vi "Save.vi"(0 "User Configuration Manager in":refnum<class "User Configuration Manager.lvclass">, 5 "Path":path, 11 "error in (no error)":errorcluster, 12 "Persistence":refnum<class "IPersist.lvclass">) -> (4 "User Configuration Manager out":refnum<class "User Configuration Manager.lvclass">, 15 "error out":errorcluster)   [LabVIEW 2017, in "User Configuration Manager.lvlib" / "User Configuration Manager.lvclass"]
doc: "Saves the manager."
uses:
  User Configuration Manager.lvclass
  <vilib>/gpm_packages/@cs/persistence/source/IPersist/IPersist.lvclass
  User Configuration Manager.lvclass/User Configuration Manager.ctl
  Accessors/Read Linked List Ref .vi
  <vilib>/gpm_packages/@cs/linked-list/Source/Linked List/ILinkedList/ILinked List.lvclass
  <vilib>/gpm_packages/@cs/linked-list/Source/Linked List/Linked List Ref/Linked List Ref.lvclass
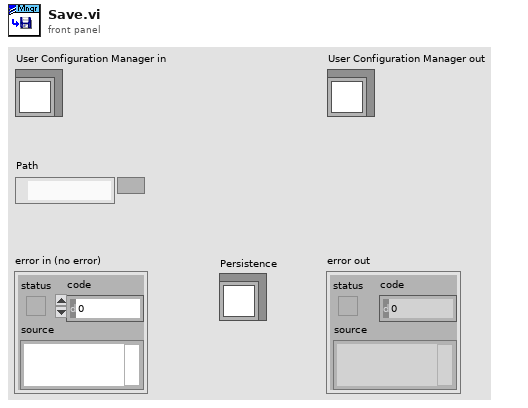
[diagram p1: front panel]
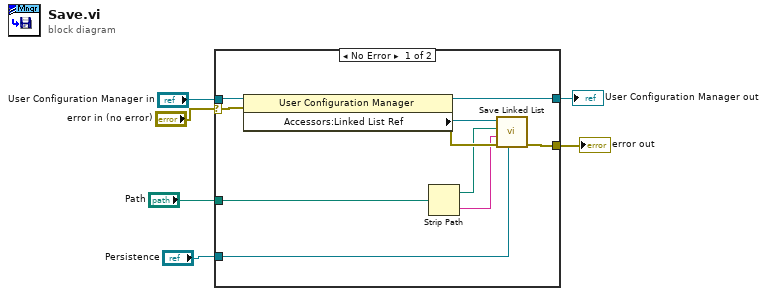
[diagram p0: block diagram]
diagram:
  n1 = case shown="No Error" "error in (no error)" {
    selector: "error in (no error)" -> [w13 w17]
    tunnel: "User Configuration Manager in" -> [w16 w18]
    tunnel: [w14 w17] -> w4
    tunnel: [w11 w18] -> w3
    tunnel: "Path" -> [w10 _]
    tunnel: "Persistence" -> [w7 _]
    frame No Error {
      n2 = property class="User Configuration Manager"(reference=w16, error in=w13) -> (reference out=w11:refnum<class "User Configuration Manager.lvclass">, error out=w12:errorcluster, "Accessors:Linked List Ref "=w15:refnum<data-value>)
      n3 = Strip Path(path=w10) -> (stripped path=w9:path, name=w8:string)
      n4 = call <vilib>:"Save Linked List.vi"("Persistence"=w7, "error in (no error)"=w12, "File Name"=w8, "Folder"=w9, "Linked List Ref"=w15) -> ("error out"=w14:errorcluster)  [unwired: 5 in, 1 out]
    }
    frame Error {
    }
  }
  "error out" <- w4
  "User Configuration Manager out" <- w3
